vi "Mask file select device.vi"(8 "Device":string, 11 "MaskFile":path=path "C:/Users/Flash/Desktop/Mask Files/SL066 Detector/SL066_mask_map_file_V3_align on D3000.csv") -> (3 "RawMask":path)   [LabVIEW 2012]
uses:
  <vilib>/Utility/file.llb/Read From Spreadsheet File (string).vi
  <vilib>/Utility/file.llb/Write To Spreadsheet File (string).vi
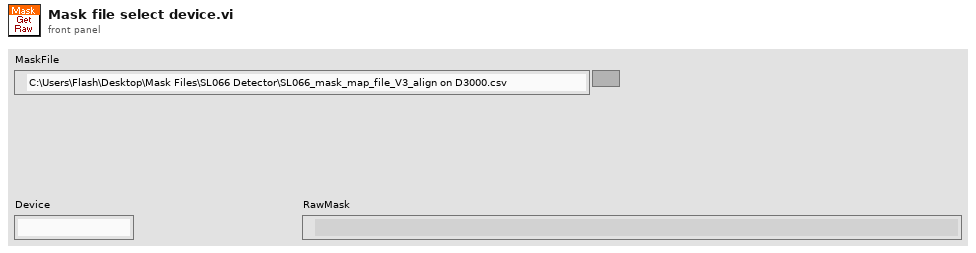
[diagram p1: front panel]
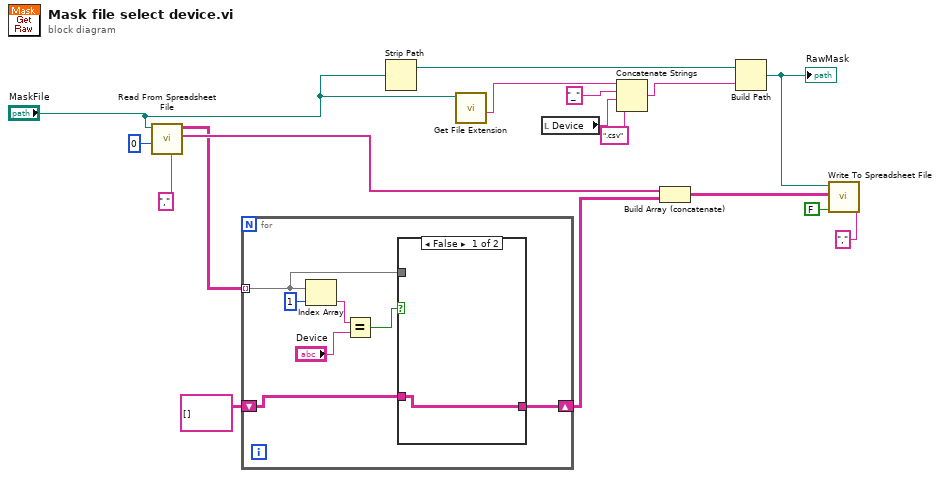
[diagram p0: block diagram]
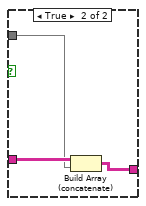
[diagram p2: hidden frame]
diagram:
  n1 = call-poly <vilib>:"Read From Spreadsheet File.vi"("delimiter (\\t)"="," ("delimiter (\\t)"), "start of read offset (chars.:0)"=0, "file path (dialog if empty)"="MaskFile") -> ("first row"=w15:string[], "all rows"=w14:string[][])  [unwired: 4 in, 3 out]
  n2 = for {
    tunnel: w14 -> [w20] mode=indexing
    shift-right: [w18] -> w3
    shift-left: string[][] [] -> [w19]
    n3 = Index Array(array=w20, index=1) -> (element=w22:string)
    n4 = Equal?(x=w22, y="Device") -> (x = y?=w21:bool)
    n5 = case shown="False" w21 {
      tunnel: w20 -> [_ w27]
      tunnel: w19 -> [w25 w28]
      tunnel: [w25 w26] -> w18
      frame False {
      }
      frame True {
        n6 = Build Array (concatenate)(w28, w27) -> (w26:string[][])
      }
    }
  }
  n7 = Strip Path(path="MaskFile") -> (stripped path=w11:path)  [unwired: 1 out]
  n8 = call <vilib>:"Get File Extension.vi"("file"="MaskFile") -> ("filename without extension"=w1:string)  [unwired: 7 in, 3 out]
  n9 = local read "Device"() -> (w12:string)
  n10 = Concatenate Strings(w1, "_" ("string"), w12, ".csv" ("string")) -> (w10:string)
  n11 = Build Array (concatenate)(w15, w3) -> (w8:string[][])
  n12 = Build Path(base path=w11, name or relative path=w10) -> (appended path=w9:path)
  "RawMask" <- w9
  n13 = call-poly <vilib>:"Write To Spreadsheet File.vi"("delimiter (\\t)"="," ("delimiter (\\t)"), "append to file? (new file:F)"=FALSE, "2D data"=w8, "file path (dialog if empty)"=w9) -> ()  [unwired: 4 in, 1 out]
